vi "Close.vi"(8 "error in (no error)":errorcluster, 11 "MelsecTCP in":refnum<class "DeltaTcp.lvclass">) -> (0 "error out":errorcluster, 3 "MelsecTCP out":refnum<class "DeltaTcp.lvclass">)   [LabVIEW 2020, in "HslCommunication.lvlib" / "DeltaTcp.lvclass"]
uses:
  DeltaTcp.lvclass
  D:/Project/Labview-Projects/General utility tool/Libraries/HslCommunication/_Dependenciecs/HslCommunication.dll
  _Dependenciecs/HslCommunication.dll
  Read reference.vi
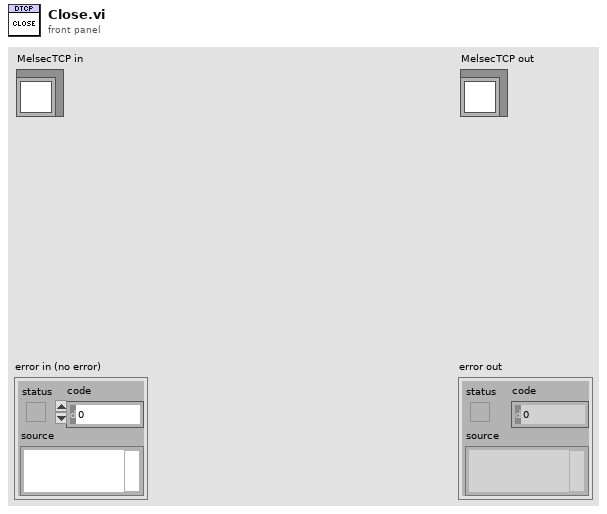
[diagram p1: front panel]
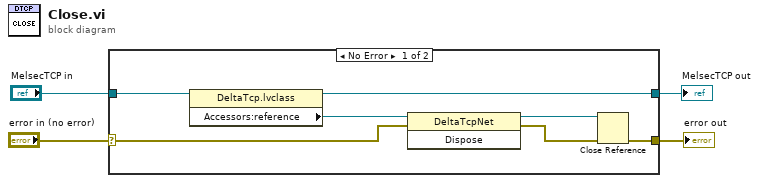
[diagram p0: block diagram]
diagram:
  n1 = case shown="No Error" "error in (no error)" {
    selector: "error in (no error)" -> [w5 w13]
    tunnel: "MelsecTCP in" -> [w11 w12]
    tunnel: [w10 w12] -> w2
    tunnel: [w9 w13] -> w1
    frame No Error {
      n2 = property class="DeltaTcp.lvclass"(reference=w11) -> (reference out=w10:refnum<class "DeltaTcp.lvclass">, "Accessors:reference"=w8:refnum<k24>)  [unwired: 1 in, 1 out]
      n3 = invoke class="DeltaTcpNet" method="Dispose"(reference=w8, error in=w5) -> (reference out=w7:refnum<k24>, error out=w6:errorcluster)  [unwired: 1 in, 1 out]
      n4 = Close Reference(reference=w7, error in (no error)=w6) -> (error out=w9:errorcluster)
    }
    frame Error {
    }
  }
  "error out" <- w1
  "MelsecTCP out" <- w2
